vi "ConfigureSimulatedCameras.vi"(8 "error in (no error)":errorcluster) -> (0 "error out":errorcluster)   [LabVIEW 2017, in "IrManageCameras.lvlib"]
uses:
  <vilib>/addons/InsightCM/Devices/Shared/Ir/IrManageCameras/IrManageCameras.lvlib
  <vilib>/addons/InsightCM/Devices/Shared/Ir/IrManageCameras/subVIs/SimConfigRefGlobal.vi
panel:
  in  "Sim Cameras":T1(array[cluster])=[{"Serial Number"="12345ABC", "Camera Type"="FLIR Ax5"}, {"Serial Number"="67890DEF", "Camera Type"="FLIR Ax5"}]
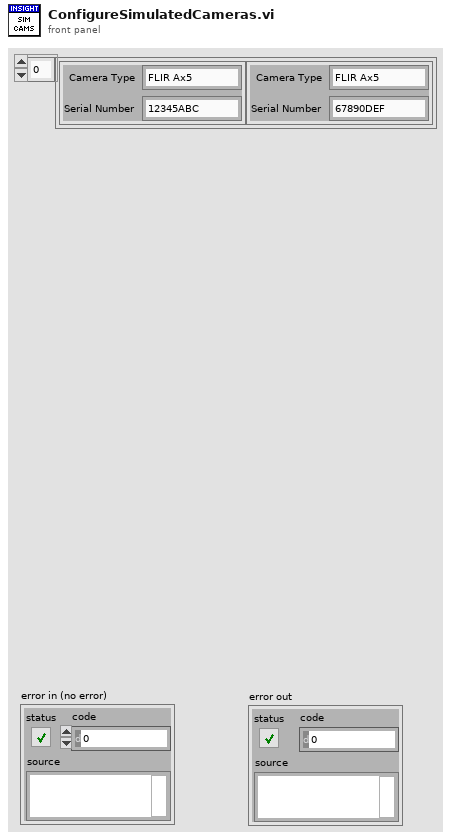
[diagram p1: front panel]
types:
  T1 = cluster{"Serial Number":string, "Camera Type":string}[]
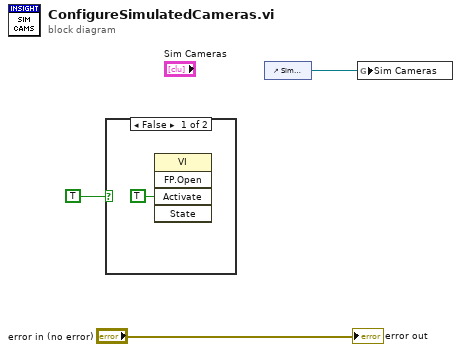
[diagram p0: block diagram]
diagram:
  n1 = case shown="False" TRUE {
    frame False {
      n2 = invoke class="VI" method="FP.Open"("Activate"=TRUE ("Activate?")) -> ()  [unwired: 4 in, 5 out]
    }
    frame True {
    }
  }
  n3 = control-ref of="Sim Cameras"() -> (w1:refnum<vi>)
  n4 = global write "SimConfigRefGlobal.vi" "Sim Cameras"(w1) -> ()
  "error out" <- "error in (no error)"
